vi "FestoCPX.Station.LaserPress.Check.vi"(8 "error in":errorcluster) -> (0 "error out":errorcluster, 1 "Work?":bool, 2 "Home?":bool)   [LabVIEW 2015]
uses:
  FestoCPX.DI.Signal.ctl
  FestoCPX.DI.Data.State.Get.vi
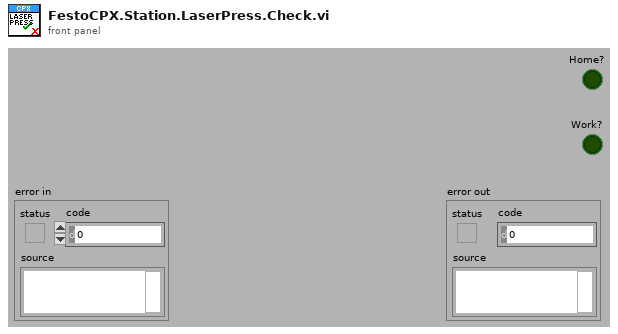
[diagram p1: front panel]
types:
  T1 = typedef "FestoCPX.DI.Signal.ctl" = enum16{"S.C. Emergency Stop", "S.C. Light Curtain", "S.C. Doors", "S.C. Table Turn", "Air Pressure 1", "Air Pressure 2", "Start Button", "White Button", "Blue Button", "Red Button", "Product present landing A", "Product present landing B", "Product present unloading A", "Product present unloading B", "Pneumatic conection's add A", "Pneumatic conection's add B", "Vent B Work", "Vent B Home", "Vent A Work", "Vent A Home", "Lock Table", "Product Press A Work", "Product Press A Home", "Product Press B Work", "Product Press B Home", "Pneumatic Connection A Work", "Pneumatic Connection A Home", "Pneumatic Connection B Work", "Pneumatic Connection B Home", "Laser Press Work", "Laser Press Home"}
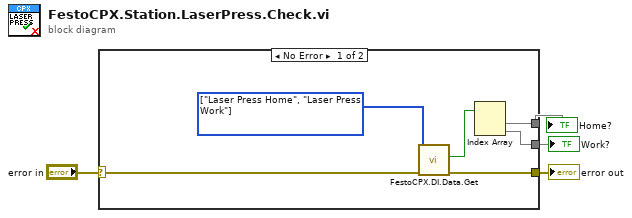
[diagram p0: block diagram]
diagram:
  n1 = case shown="No Error" "error in" {
    selector: "error in" -> [w8 w11]
    tunnel: [w7 w11] -> w4
    tunnel: [w10 _] -> w2
    tunnel: [w9 _] -> w1
    frame No Error {
      w5 = T1[] [enum."Laser Press Home", enum."Laser Press Work"] items=["S.C. Emergency Stop", "S.C. Light Curtain", "S.C. Doors", "S.C. Table Turn", "Air Pressure 1", "Air Pressure 2", "Start Button", "White Button", "Blue Button", "Red Button", "Product present landing A", "Product present landing B", "Product present unloading A", "Product present unloading B", "Pneumatic conection's add A", "Pneumatic conection's add B", "Vent B Work", "Vent B Home", "Vent A Work", "Vent A Home", "Lock Table", "Product Press A Work", "Product Press A Home", "Product Press B Work", "Product Press B Home", "Pneumatic Connection A Work", "Pneumatic Connection A Home", "Pneumatic Connection B Work", "Pneumatic Connection B Home", "Laser Press Work", "Laser Press Home"]
      n2 = call-poly "FestoCPX.DI.Data.Get.vi"("error in (no error)"=w8, "CPX.DI"=w5) -> ("error out"=w7:errorcluster, "State"=w6:bool)  [unwired: 8 in]
      n3 = Index Array(array=w6) -> (element #1=w10, element #2=w9)  [unwired: 2 in]
    }
    frame Error {
    }
  }
  "error out" <- w4
  "Home?" <- w2
  "Work?" <- w1
